vi "Create All Message Queues.vi"(8 "error in (no error)":errorcluster) -> (0 "error out":errorcluster, 3 "Message Queues out":T1)   [LabVIEW 2020, in "Omega Platinum Series Plugin.lvlib" / "Message Queue.lvlib"]
doc: "This VI creates and initializes all the message queues for your application. If your application requires more than one message queue, right-click the \"Message Queues\" constant above and select Open Type Def. Add the new Message Queue(s) to the type definition, then initialize them in this VI."
uses:
  Message Queue.lvlib
  All Message Queues.ctl
  Message Cluster.ctl
  Enqueue Message (Single).vi
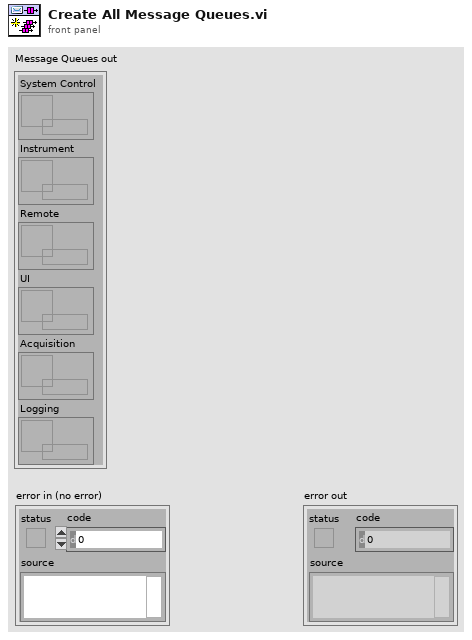
[diagram p1: front panel]
types:
  T1 = typedef "Omega Platinum Series Plugin.lvlib/Message Queue.lvlib/All Message Queues.ctl" = cluster{"System Control":refnum<queue>, "Instrument":refnum<queue>, "Remote":refnum<queue>, "UI":refnum<queue>, "Acquisition":refnum<queue>, "Logging":refnum<queue>}
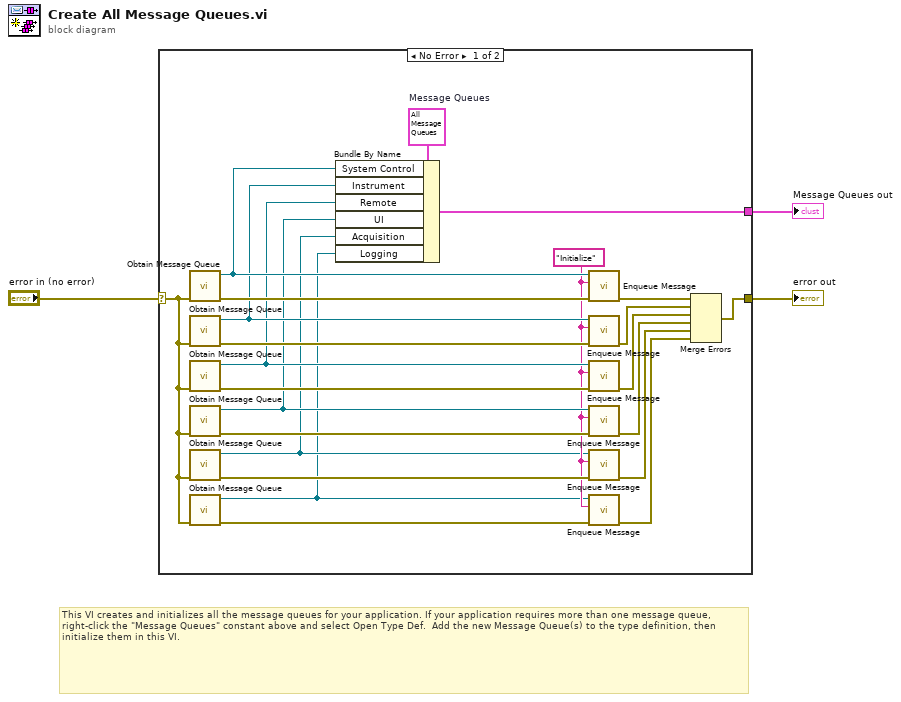
[diagram p0: block diagram]
diagram:
  # "This VI creates and initializes all the message queues for your application. If your application requires more than one message queue, right-click the \"Message Queues\" constant above and select Open Type Def.  Add the new Message Queue(s) to the type definition, then initialize them in this VI."
  n1 = case shown="No Error" "error in (no error)" {
    selector: "error in (no error)" -> [w8 w27]
    tunnel: [w19 w27] -> w3
    tunnel: [w24 _] -> w2
    frame No Error {
      w9 = "Initialize" ("Message")
      w25 = T1 {"System Control"=refnum, "Instrument"=refnum, "Remote"=refnum, "UI"=refnum, "Acquisition"=refnum, "Logging"=refnum}  # Message Queues
      n2 = call "Obtain Message Queue.vi"("error in (no error)"=w8) -> ("error out"=w23:errorcluster, "Message Queue"=w22:refnum<queue>)  [unwired: 9 in]
      n3 = call "Obtain Message Queue.vi"("error in (no error)"=w8) -> ("error out"=w21:errorcluster, "Message Queue"=w20:refnum<queue>)  [unwired: 9 in]
      n4 = call "Obtain Message Queue.vi"("error in (no error)"=w8) -> ("error out"=w17:errorcluster, "Message Queue"=w16:refnum<queue>)  [unwired: 9 in]
      n5 = call "Obtain Message Queue.vi"("error in (no error)"=w8) -> ("error out"=w15:errorcluster, "Message Queue"=w14:refnum<queue>)  [unwired: 9 in]
      n6 = call "Obtain Message Queue.vi"("error in (no error)"=w8) -> ("error out"=w11:errorcluster, "Message Queue"=w7:refnum<queue>)  [unwired: 9 in]
      n7 = call "Obtain Message Queue.vi"("error in (no error)"=w8) -> ("error out"=w10:errorcluster, "Message Queue"=w6:refnum<queue>)  [unwired: 9 in]
      n8 = Bundle By Name(cluster=w25, "System Control"=w22, "Instrument"=w20, "Remote"=w16, "UI"=w14, "Acquisition"=w7, "Logging"=w6) -> (w24:T1)
      n9 = call-poly "Enqueue Message.vi"("error in (no error)"=w23, "Message"=w9, "Message Queue"=w22) -> ("error out"=w26:errorcluster)  [unwired: 7 in, 1 out]
      n10 = call-poly "Enqueue Message.vi"("error in (no error)"=w21, "Message"=w9, "Message Queue"=w20) -> ("error out"=w18:errorcluster)  [unwired: 7 in, 1 out]
      n11 = call-poly "Enqueue Message.vi"("error in (no error)"=w17, "Message"=w9, "Message Queue"=w16) -> ("error out"=w13:errorcluster)  [unwired: 7 in, 1 out]
      n12 = call-poly "Enqueue Message.vi"("error in (no error)"=w15, "Message"=w9, "Message Queue"=w14) -> ("error out"=w12:errorcluster)  [unwired: 7 in, 1 out]
      n13 = call-poly "Enqueue Message.vi"("error in (no error)"=w11, "Message"=w9, "Message Queue"=w7) -> ("error out"=w5:errorcluster)  [unwired: 7 in, 1 out]
      n14 = call-poly "Enqueue Message.vi"("error in (no error)"=w10, "Message"=w9, "Message Queue"=w6) -> ("error out"=w4:errorcluster)  [unwired: 7 in, 1 out]
      n15 = Merge Errors(w26, w18, w13, w12, w5, w4) -> (w19:errorcluster)
    }
    frame Error {
    }
  }
  "Message Queues out" <- w2
  "error out" <- w3
